vi "SDI-12 Single Operation.vi"(0 "RS232 Port In":refnum<visa-resource-name>="COM11", 5 "Sensor Address In":string="0", 7 "Cumulative Volume":dbl, 11 "Error In (No Error)":errorcluster, 12 "Initialize/Close?":bool=TRUE) -> (4 "RS232 Port Out":refnum<visa-resource-name>, 6 "Address Out":string="a" caption="sensor address out", 8 "Cluster":T1, 13 "Measurements Out":dbl[](array[numeric]), 15 "Error Out":errorcluster)   [LabVIEW 2016]
doc: "A general set of examples of the SDI-12 API for a generic sensor. A tab control separates each example, and contains the following examples:\n1. Read Single.\n2. Read Multiple.\n3. Acknowledge Active.\n4. Change Address.\n5. Address Query.\n6. Send Identification."
uses:
  SDI-12/SDI-12.lvlib
panel:
  out "Battery Voltage (V)":dbl
  out "End time":timestamp
  out "Number of Measurements Out":i32
  in  "Measurement Type In (Normal)":i32(ring)=1 items=["Normal", "Concurrent", "Continuous"]
  out "Parameter Out":i32(ring) items=["0", "1", "2", "3", "4", "5", "6", "7", "8", "9"]
  in  "Parameter In (0)":i32(ring) items=["0", "1", "2", "3", "4", "5", "6", "7", "8", "9"]
  in  "CRC (False)":bool
  out "CRC Out":bool
  out "Measurement Type Out":i32(ring) items=["Normal", "Concurrent", "Continuous"]
  out "Time (s)":dbl
  out "start time":timestamp
  # "deg C"
  # "pH"
  # "specific conductance"
  # "salinity"
  # "DO % saturation"
  # "DO mg/L"
  # "ORP"
  # "depth"
  # "battery"
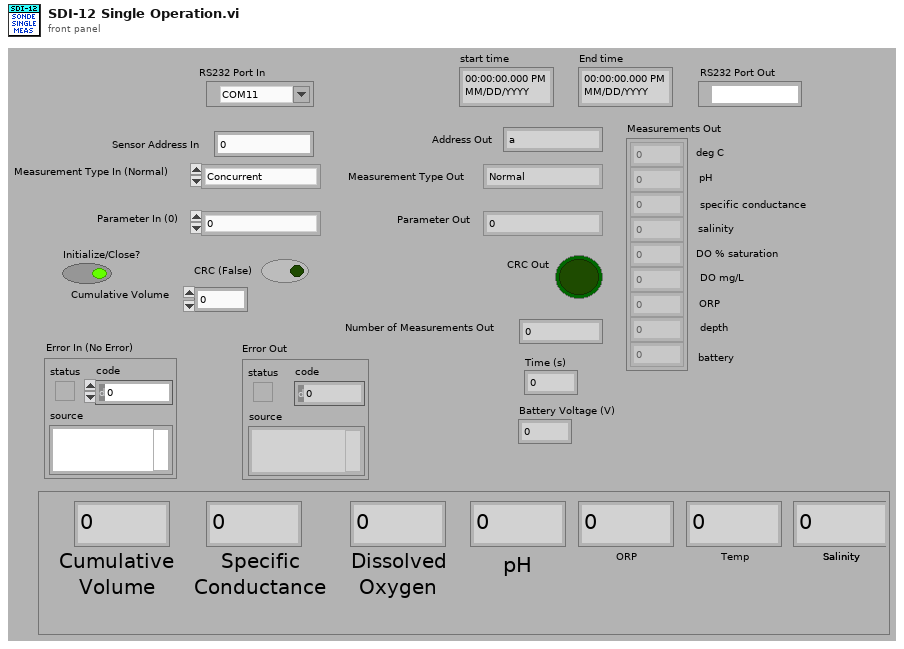
[diagram p1: front panel]
types:
  T1 = cluster{"Cumulative\nVolume":dbl, "Specific\nConductance":dbl, "Dissolved\nOxygen":dbl, "pH":dbl, "ORP":dbl, "Temp":dbl, "Salinity":dbl}
  T2 = typedef "sonde cluster.ctl" = cluster{"Cumulative\nVolume (ml)":dbl, "Specific\nCond (mS)":dbl, "Dissolved\nOxygen mg/L":dbl, "pH":dbl, "ORP":dbl, "Temp\ndeg C":dbl, "Salinity":dbl}
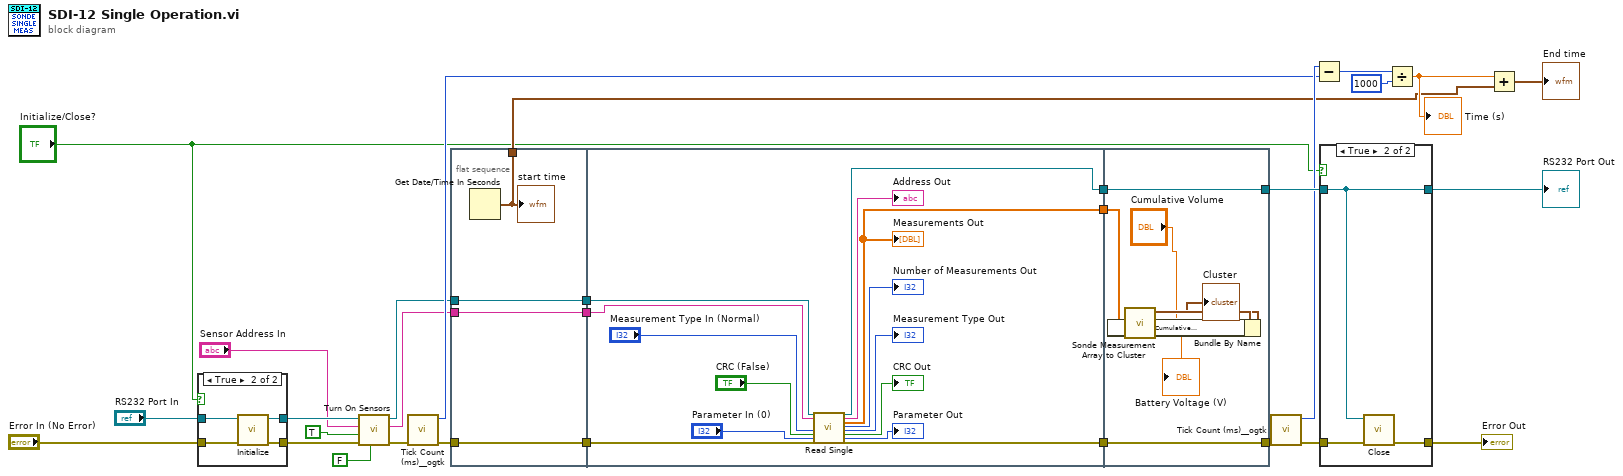
[diagram p0: block diagram]
diagram:
  n1 = case shown="True" "Initialize/Close?" {
    tunnel: "RS232 Port In" -> [w32 w36]
    tunnel: "Error In (No Error)" -> [w31 w35]
    tunnel: [w31 w34] -> w10
    tunnel: [w32 w33] -> w8
    frame False {
    }
    frame True {
      n2 = call "Initialize.vi"("Error In (No Error)"=w35, "RS232 Port In"=w36) -> ("Error Out"=w34:errorcluster, "RS232 Port Out"=w33:refnum<visa-resource-name>)  [unwired: 8 in]
    }
  }
  n3 = call "Turn On Sensors.vi"("Initialize/Close?"=FALSE, "Error In (No Error)"=w10, "Sensor On/Off"=TRUE, "Sensor Address In"="Sensor Address In", "RS232 Port In"=w8) -> ("Error Out"=w9:errorcluster, "Address Out"=w5:string, "RS232 Port Out"=w7:refnum<visa-resource-name>)  [unwired: 3 in, 1 out]
  n4 = call "Tick Count (ms)__ogtk.vi"("error in (no error)"=w9) -> ("error out"=w24:errorcluster, "millisecond timer value"=w22:u32)  [unwired: 9 in]
  n5 = flat-sequence {
    tunnel: w5 -> [w38]
    tunnel: w7 -> [w39]
    tunnel: w24 -> [w40]
    tunnel: [w40] -> w17
    tunnel: [w39] -> w16
    tunnel: [w38] -> w15
    tunnel: [w37] -> w14
    tunnel: w17 -> [w44]
    tunnel: w16 -> [w43]
    tunnel: w15 -> [w41]
    tunnel: [w54] -> w13
    tunnel: [w53] -> w12
    tunnel: [w42] -> w11
    tunnel: [w60] -> w25
    tunnel: [w61] -> w27
    tunnel: w13 -> [w61]
    tunnel: w12 -> [w60]
    tunnel: w11 -> [w59]
    frame #0 {
      n6 = Get Date/Time In Seconds() -> (seconds since 1Jan1904=w37:timestamp)
      "start time" <- w37
    }
    frame #1 {
      n7 = call "Read Single.vi"("RS232 Port In"=w43, "Sensor Address In"=w41, "Measurement Type In (Normal)"="Measurement Type In (Normal)", "CRC (False)"="CRC (False)", "Parameter In (0)"="Parameter In (0)", "Error In (No Error)"=w44) -> ("RS232 Port Out"=w54:refnum<visa-resource-name>, "Sensor Address Out"=→"Address Out":string, "Measurements Out"=w42:dbl[], "Number of Measurements Out"=→"Number of Measurements Out":i32, "Measurement Type Out"=→"Measurement Type Out":i32, "CRC Out"=→"CRC Out":bool, "Parameter Out"=→"Parameter Out":i32, "Error Out"=w53:errorcluster)  [unwired: 14 in]
      "Measurements Out" <- w42
    }
    frame #2 {
      n8 = call "Sonde Measurement Array to Cluster.vi"("Measurements In"=w59) -> ("Battery Voltage (V)"=→"Battery Voltage (V)":dbl, "Sonde Data Cluster"=w58:T2)  [unwired: 9 in]
      n9 = Bundle By Name(cluster=w58, "Cumulative\nVolume (ml)"="Cumulative Volume") -> (→"Cluster":T2)
    }
  }
  n10 = call "Tick Count (ms)__ogtk.vi"("error in (no error)"=w25) -> ("error out"=w28:errorcluster, "millisecond timer value"=w23:u32)  [unwired: 9 in]
  n11 = Subtract(x=w23, y=w22) -> (x-y=w21:u32)
  n12 = case shown="True" "Initialize/Close?" {
    tunnel: w28 -> [w63 w66]
    tunnel: w27 -> [w62 w64]
    tunnel: [w63 w65] -> w26
    tunnel: [w62 w64] -> w2
    frame False {
    }
    frame True {
      n13 = call "Close.vi"("Error In (No Error)"=w66, "RS232 Port In"=w64) -> ("Error Out"=w65:errorcluster)  [unwired: 9 in]
    }
  }
  "Error Out" <- w26
  "RS232 Port Out" <- w2
  n14 = Divide(x=w21, y=u32 1000) -> (x/y=w19:dbl)
  "Time (s)" <- w19
  n15 = Add(x=w19, y=w14) -> (x+y=→"End time":timestamp)
